vi "rod_oscillation_V1.vi"() -> ()   [LabVIEW 2012]
uses:
  <vilib>/Motion/FlexMotion/CustomControls/CustomControls.llb/Axis To Control.flx
  <vilib>/Motion/FlexMotion/FunctionsVIs/Trajectory.llb/Load Accel/Decel in RPS/sec.flx
  <vilib>/Motion/FlexMotion/FunctionsVIs/StartStopMotion.llb/Start Motion (8 axes).flx
  <vilib>/Motion/FlexMotion/FunctionsVIs/StartStopMotion.llb/Stop Motion (8 axes).flx
  <vilib>/measure/NI_MABase.lvlib
panel:
  in  "#  samples/cycle":dbl=300.0
  in  "Mean RPM":dbl=200.0 format="%0.2p"
  in  "#  of cycles":dbl=100.0
  out "dt (ms)":dbl
  in  "amplitude RPM":dbl=200.0 format="%0.2p"
  in  "frequency (Hz)":dbl=5.0 format="%0.2p"
  in  "stop":bool
  in  "Acceleration Limit (RPS/s)":dbl=20.0 min=0.0 format="%.2f"
  in  "Board ID":T1=1 min=1 max=32 step=1
  in  "Axis":T2=1 items=["Axis 1"=1, "Axis 2"=2, "Axis 3"=3, "Axis 4"=4, "Axis 5"=5, "Axis 6"=6, "Axis 7"=7, "Axis 8"=8]
  out "Velocity":cluster{dbl, dbl, dbl[]}(graph)
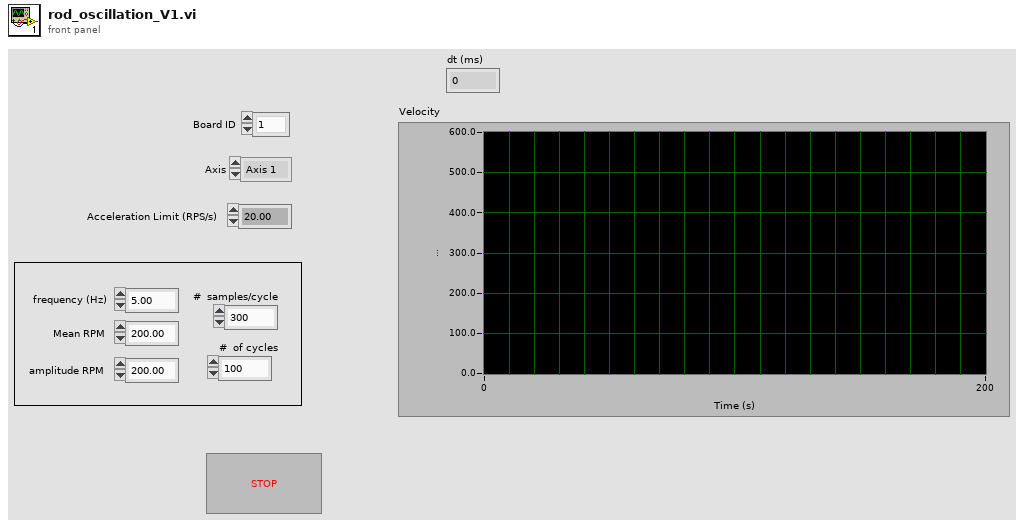
[diagram p1: front panel]
types:
  T1 = typedef "Board Id" = u8
  T2 = typedef "Axis To Control.flx" = u16
  T3 = enum16{"Absolute Position", "Relative Position", "Velocity", "Relative to Cap Pos", "Modulus Position", "Absolute Contouring", "Relative Contouring"}
  T4 = typedef "Bd Id Out" = u8
  T5 = typedef "Resource Out (Enum).flx" = u16
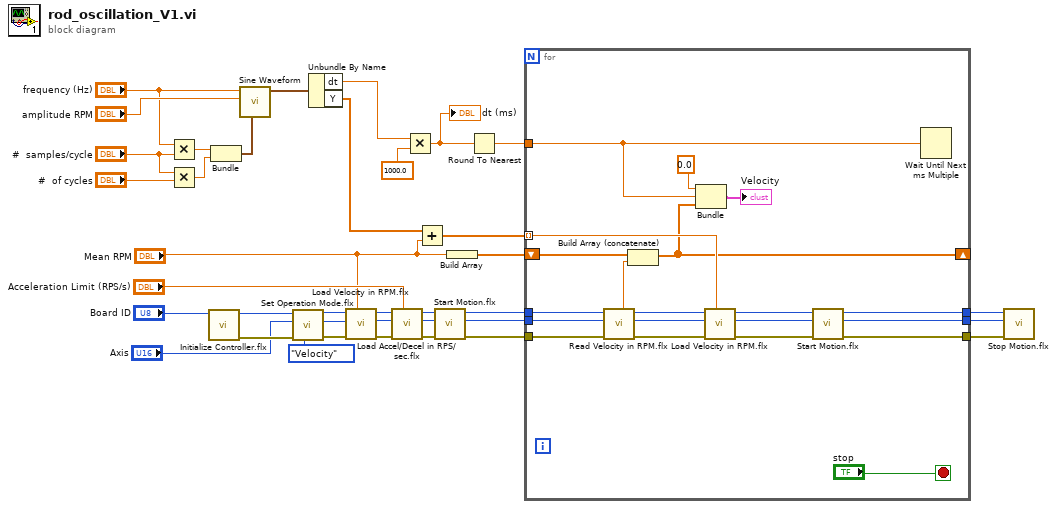
[diagram p0: block diagram]
diagram:
  n1 = Multiply(x="frequency (Hz)", y="#  samples/cycle") -> (x*y=w7:dbl)
  n2 = Multiply(x="#  samples/cycle", y="#  of cycles") -> (x*y=w6:dbl)
  n3 = call <vilib>:"Initialize Controller.flx"("Board ID"="Board ID") -> ("error out"=w3:errorcluster, "Bd ID Out"=w2:T4)  [unwired: 7 in]
  n4 = Bundle(w7, w6) -> (w5:cluster{dbl, dbl})  [unwired: 1 in]
  n5 = call <vilib>:"Sine Waveform.vi"("sampling info"=w5, "amplitude"="amplitude RPM", "frequency"="frequency (Hz)") -> ("signal out"=w19:waveform(dbl))  [unwired: 7 in, 1 out]
  n6 = call <vilib>:"Set Operation Mode.flx"("Position Mode (Absolute)"=T3."Velocity", "error in (no error)"=w3, "Axis or Vector Space"="Axis", "Board ID"=w2) -> ("error out"=w25:errorcluster, "Resource Output"=w26:T5, "Bd ID Out"=w27:T4)  [unwired: 2 in]
  n7 = Unbundle By Name(w19) -> ("dt"=w14:dbl, "Y"=w15:dbl[])
  n8 = call <vilib>:"Load Velocity in RPM.flx"("Velocity (500)"="Mean RPM", "error in (no error)"=w25, "Axis or Vector Space"=w26, "Board ID"=w27) -> ("error out"=w31:errorcluster, "Resource Output"=w30:T5, "Bd ID Out"=w29:T4)  [unwired: 3 in]
  n9 = call "Load Accel/Decel in RPS/sec.flx"("Value (200)"="Acceleration Limit (RPS/s)", "error in (no error)"=w31, "Axis or Vector Space"=w30, "Board ID"=w29) -> ("error out"=w34:errorcluster, "Resource Output"=w33:T5, "Bd ID Out"=w32:T4)  [unwired: 3 in]
  n10 = Multiply(x=w14, y=1000.0) -> (x*y=w12:dbl)
  "dt (ms)" <- w12
  n11 = Add(x=w15, y="Mean RPM") -> (x+y=w17:dbl[])
  n12 = call-poly <vilib>:"Start Motion.flx"("error in (no error)"=w34, "Axis or Vector Space"=w33, "Board ID"=w32) -> ("error out"=w37:errorcluster, "Resource Output"=w36:T5, "Bd ID Out"=w35:T4)  [unwired: 3 in]
  n13 = Build Array("Mean RPM") -> (w16:dbl[])
  n14 = Round To Nearest(number=w12) -> (nearest integer value=w18:dbl)
  n15 = for {
    tunnel: [w49] -> w22
    tunnel: [w50] -> w23
    tunnel: [w51] -> w24
    tunnel: w37 -> [w52]
    tunnel: w36 -> [w53]
    tunnel: w35 -> [w54]
    tunnel: w18 -> [w44]
    shift-right: [w38] -> _
    shift-left: w16 -> [w41]
    tunnel: w17 -> [w39] mode=indexing
    stop <- "stop" stop-if-true
    n16 = call <vilib>:"Read Velocity in RPM.flx"("error in (no error)"=w52, "Axis or Vector Space"=w53, "Board ID"=w54) -> ("error out"=w50:errorcluster, "Resource Output"=w49:T5, "Bd ID Out"=w51:T4, "Filtered Velocity"=w40:dbl)  [unwired: 3 in]
    n17 = Build Array (concatenate)(w41, w40) -> (w38:dbl[])
    n18 = Bundle(0.0, w44, w38) -> (→"Velocity":cluster{dbl, dbl, dbl[]})  [unwired: 1 in]
    n19 = call <vilib>:"Load Velocity in RPM.flx"("Velocity (500)"=w39, "error in (no error)"=w50, "Axis or Vector Space"=w49, "Board ID"=w51) -> ("error out"=w48:errorcluster, "Resource Output"=w47:T5, "Bd ID Out"=w46:T4)  [unwired: 3 in]
    n20 = call-poly <vilib>:"Start Motion.flx"("error in (no error)"=w48, "Axis or Vector Space"=w47, "Board ID"=w46) -> ()  [unwired: 3 in, 3 out]
    n21 = Wait Until Next ms Multiple(millisecond multiple=w44) -> ()  [unwired: 1 out]
  }
  n22 = call-poly <vilib>:"Stop Motion.flx"("error in (no error)"=w23, "Axis or Vector Space"=w22, "Board ID"=w24) -> ()  [unwired: 4 in, 3 out]
